vi "Update UI Data.vi"(0 "DAQ in":refnum<class "DAQ.lvclass">, 5 "QPD Voltage X":dbl format="%#_13g", 7 "QPD Voltage Y":dbl format="%#_13g", 9 "QPD  Sum":dbl format="%#_13g", 11 "error in (no error)":errorcluster) -> (4 "DAQ out":refnum<class "DAQ.lvclass">, 15 "error out":errorcluster)   [LabVIEW 2020, in "DAQ.lvlib" / "DAQ.lvclass"]
uses:
  DAQ.lvclass
  DAQ.lvclass/DAQ.ctl
  DAQ Controller Messages/Update UI Msg/Update UI Msg.lvclass/Update UI Msg.ctl
  <vilib>/ActorFramework/Message Enqueuer/Message Enqueuer.lvclass/Message Enqueuer.ctl
  <vilib>/ActorFramework/Message Enqueuer/Enqueue.vi
  DAQ Controller Messages/Update UI Msg/Update UI Msg.lvclass
  C:/Program Files/National Instruments/LabVIEW 2020/vi.lib/ActorFramework/Message/Message.lvclass
  <vilib>/ActorFramework/Message Priority Queue/Priority Enqueue.vi
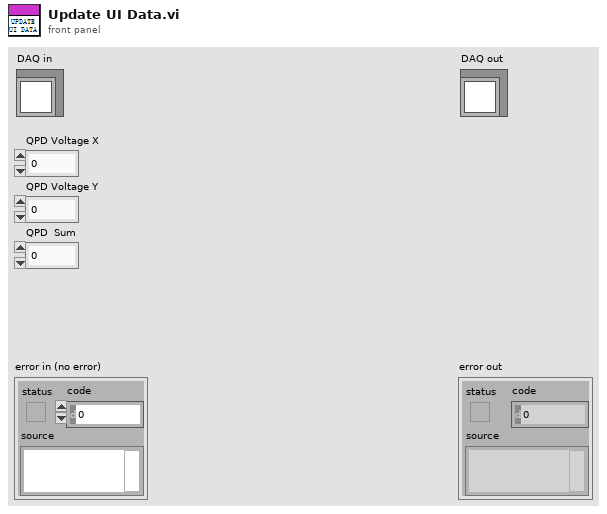
[diagram p1: front panel]
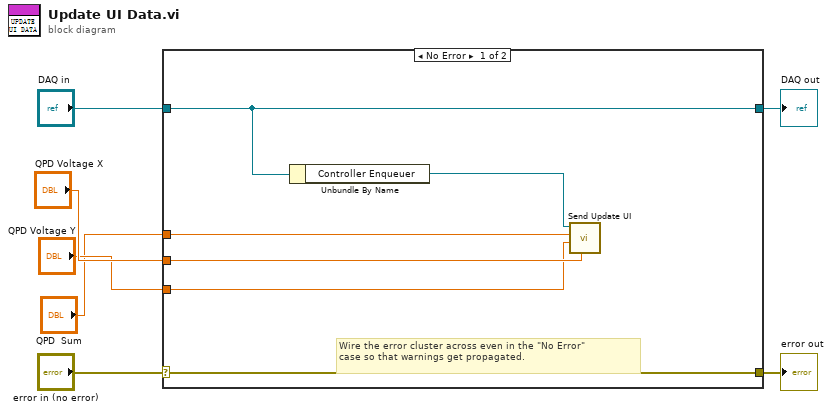
[diagram p0: block diagram]
diagram:
  n1 = case shown="No Error" "error in (no error)" {
    selector: "error in (no error)" -> [w13 w15]
    tunnel: [w13 w15] -> w6
    tunnel: [w12 w14] -> w4
    tunnel: "DAQ in" -> [w12 w14]
    tunnel: "QPD Voltage X" -> [w10 _]
    tunnel: "QPD Voltage Y" -> [w9 _]
    tunnel: "QPD  Sum" -> [w8 _]
    frame No Error {
      # "Wire the error cluster across even in the \"No Error\"\ncase so that warnings get propagated."
      n2 = Unbundle By Name(w12) -> ("Controller Enqueuer"=w11:refnum<class "Message Enqueuer.lvclass">)
      n3 = call "Send Update UI.vi"("QPD Voltage X"=w10, "QPD Voltage Y"=w9, "QPD  Sum"=w8, "Message Enqueuer"=w11) -> ()  [unwired: 6 in, 2 out]
    }
    frame Error {
    }
  }
  "error out" <- w6
  "DAQ out" <- w4
